vi "Create File.vi"(8 "error in":errorcluster, 11 "Path":refnum<class "UTF-8 Path.lvclass">) -> (0 "error out":errorcluster, 2 "result":i32, 3 "Path dup":refnum<class "UTF-8 Path.lvclass">)   [LabVIEW 2020, in "G-Unicode.lvlib"]
doc: "Create a file on disk at the specified path. To be used in conjunction with Path to Shortname.vi."
uses:
  G-Unicode.lvlib
  Types/UTF-8 Path/UTF-8 Path.lvclass
  Types/UTF-8 Path/UTF-8 Path.lvclass/UTF-8 Path.ctl
  7c1cad48-502a-40d5-8bcd-fa57563fefc2.vi
  Types/UTF-8 Path/Read Raw UTF-8 Path.vi
  lib/g_unicode_32.dll
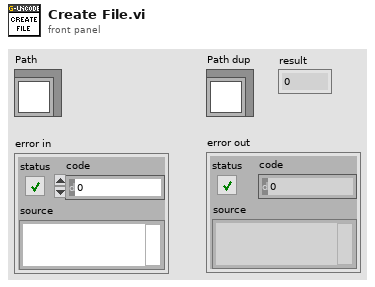
[diagram p1: front panel]
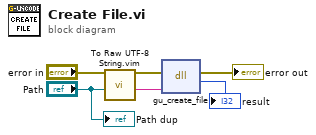
[diagram p0: block diagram]
diagram:
  n1 = call "To Raw UTF-8 String.vim"("error in"="error in", "Data"="Path") -> ("Raw UTF-8 String"=w5:string, "error out"=w3:errorcluster)  [unwired: 8 in]
  n2 = dll-call lib="C:/github/dataflowg/g-unicode/src/LabVIEW/G-Unicode/lib/g_unicode_*.*" fn="gu_create_file"(error in=w3, "utf8_path"=w5) -> (error out=→"error out":errorcluster, "result"=→"result":i32)  [unwired: 3 in, 1 out]
  "Path dup" <- "Path"
